vi "RagetoCellid.vi"(11 "Voltage ID Range":string) -> (0 "Error out":errorcluster, 3 "Cell ids":string[](array[string]))   [LabVIEW 2026]
uses:
  6e724493-33b7-456a-99ad-c74c3a75b991.vi
  <vilib>/regexp/Match Regular Expression.xnode
panel:
  out "whole match":string
  # "Used to put a str to induvidual cell id"
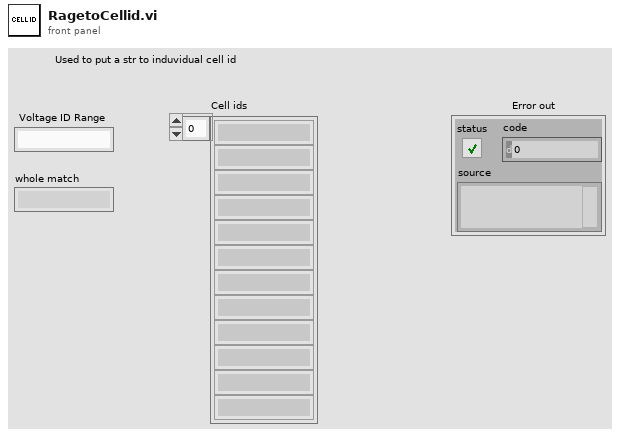
[diagram p1: front panel]
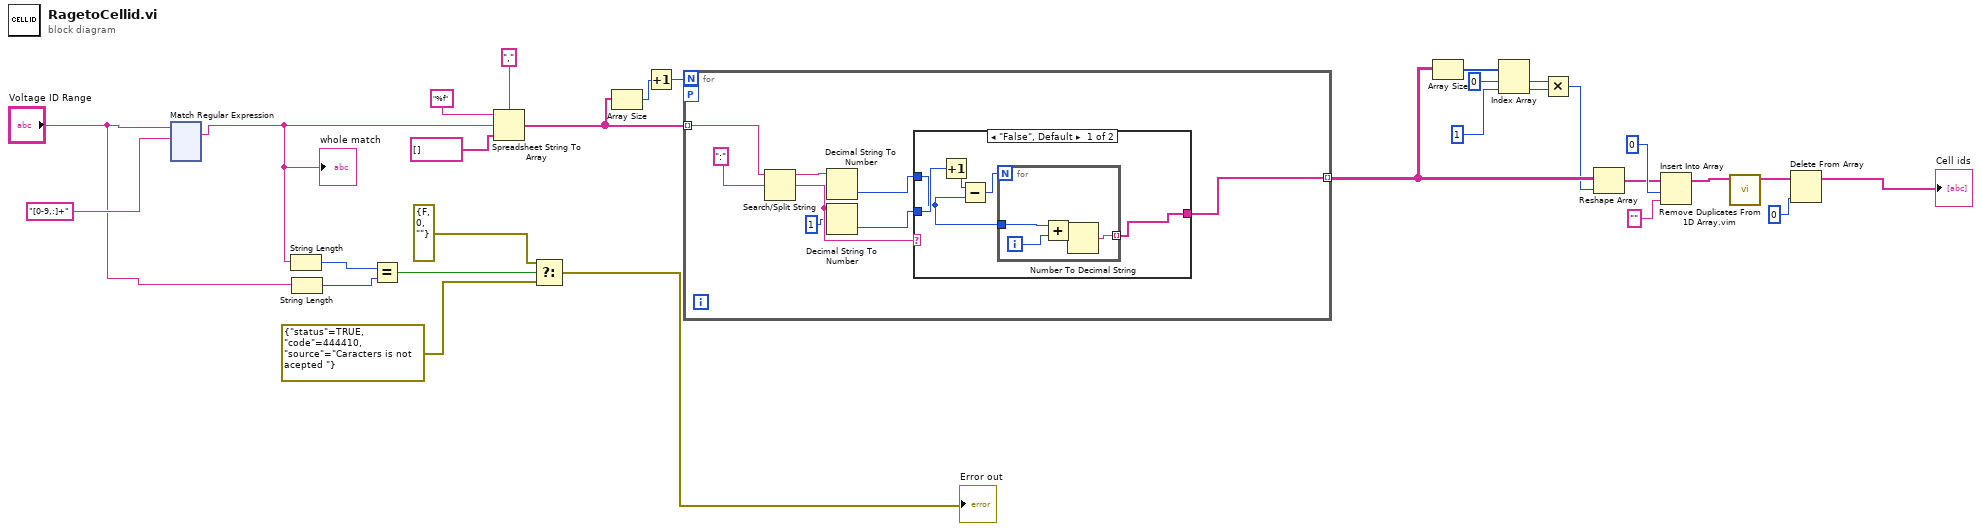
[diagram p0: block diagram]
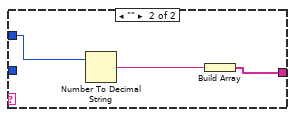
[diagram p2: hidden frame]
diagram:
  n1 = xnode "Match Regular Expression"("input string"="Voltage ID Range", "regular expression"="[0-9,:]+") -> ("whole match"=w4:string)  [unwired: 4 in, 4 out]
  "whole match" <- w4
  n2 = String Length(string=w4) -> (length=w3:i32)
  n3 = String Length(string="Voltage ID Range") -> (length=w2:i32)
  n4 = Equal?(x=w3, y=w2) -> (x = y?=w8:bool)
  n5 = Spreadsheet String To Array(delimiter (Tab)="," ("format string"), format string="%f", spreadsheet string=w4, array type (2D Dbl)=string[] []) -> (array=w11:string[])
  n6 = Select(t=errorcluster {"status"=FALSE, "code"=0, "source"=""}, s=w8, f=errorcluster {"status"=TRUE, "code"=444410, "source"="Caracters is not acepted "} ("error constant")) -> (s? t:f=→"Error out":errorcluster)
  n7 = Array Size(array=w11) -> (size(s)=w15:i32)
  n8 = Increment(x=w15) -> (x+1=w16:i32)
  n9 = for {
    N: w16 -> [_]
    workers-P: _ -> [_]
    tunnel: [w32] -> w29 mode=indexing
    tunnel: w11 -> [w30] mode=indexing
    n10 = Search/Split String(string=w30, search string/char (-)=":") -> (substring before match=w37:string, match + rest of string=w36:string)  [unwired: 1 in, 1 out]
    n11 = Decimal String To Number(string=w37) -> (number=w35:i32)  [unwired: 2 in, 1 out]
    n12 = Decimal String To Number(string=w36, offset=1) -> (number=w34:i32)  [unwired: 1 in, 1 out]
    n13 = case shown="\"False\", Default" w36 {
      tunnel: w35 -> [w38 w49]
      tunnel: w34 -> [w40 _]
      tunnel: [w41 w47] -> w32
      frame "False", Default {
        n14 = Increment(x=w40) -> (x+1=w39:i32)
        n15 = Subtract(x=w39, y=w38) -> (x-y=w42:i32)
        n16 = for {
          N: w42 -> [_]
          tunnel: w38 -> [w46]
          tunnel: [w43] -> w41 mode=indexing
          i -> [w45]
          n17 = Add(x=w46, y=w45) -> (x+y=w44:i32)
          n18 = Number To Decimal String(number=w44) -> (decimal integer string=w43:string)  [unwired: 1 in]
        }
      }
      frame "" {
        n19 = Number To Decimal String(number=w49) -> (decimal integer string=w48:string)  [unwired: 1 in]
        n20 = Build Array(w48) -> (w47:string[])
      }
    }
  }
  n21 = Array Size(array=w29) -> (size(s)=w17:i32[])
  n22 = Index Array(array=w17, index #1=0 ("index"), index #2=1 ("index")) -> (element #1=w21:i32, element #2=w20:i32)
  n23 = Multiply(x=w21, y=w20) -> (x*y=w22:i32)
  n24 = Reshape Array(w29, w22) -> (w23:string[])
  n25 = Insert Into Array(array=w23, index=0, new element="" ("new element/subarray")) -> (w24:string[])
  n26 = call "Remove Duplicates From 1D Array.vim"("array"=w24) -> ("array with duplicates removed"=w27:string[])  [unwired: 10 in]
  n27 = Delete From Array(array=w27, index=0) -> (array with subset deleted=→"Cell ids":string[])  [unwired: 1 in, 1 out]
